vi "MsgSetTemp.vi"   [LabVIEW 2018]
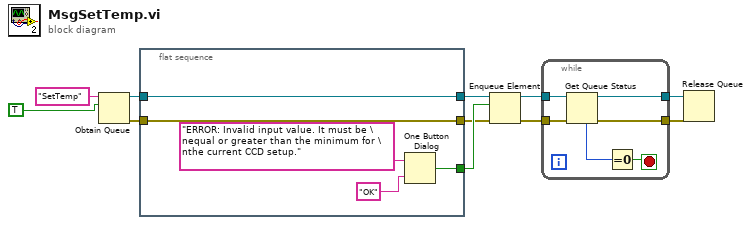
[diagram p0: block diagram]
diagram:
  n1 = Obtain Queue(name (unnamed)="SetTemp", element data type=TRUE) -> (queue out=w9:refnum<queue>, error out=w6:errorcluster)  [unwired: 3 in, 1 out]
  n2 = flat-sequence {
    tunnel: w9 -> [w15]
    tunnel: [w15] -> w8
    tunnel: [w14] -> w7
    tunnel: [w13] -> w5
    tunnel: w6 -> [w13]
    frame #0 {
      n3 = One Button Dialog(message="ERROR: Invalid input value. It must be \nequal or greater than the minimum for \nthe current CCD setup.", button name ("OK")="OK" ("T button name (\"OK\")")) -> (true=w14:bool)
    }
  }
  n4 = Enqueue Element(queue=w8, element=w7, error in (no error)=w5) -> (queue out=w4:refnum<queue>, error out=w3:errorcluster)  [unwired: 1 in, 1 out]
  n5 = while {
    tunnel: w4 -> [w22]
    tunnel: w3 -> [w21]
    tunnel: [w20] -> w2
    tunnel: [w19] -> w1
    stop <- w18 stop-if-true
    n6 = Get Queue Status(queue=w22, error in (no error)=w21) -> (queue out=w20:refnum<queue>, error out=w19:errorcluster, # elements in queue=w17:i32)  [unwired: 1 in, 5 out]
    n7 = Equal To 0?(x=w17) -> (x = 0?=w18:bool)
  }
  n8 = Release Queue(queue=w2, error in (no error)=w1) -> ()  [unwired: 1 in, 3 out]
